vi "20170425-lecture4-1 string.vi"() -> ()   [LabVIEW 2014]
panel:
  out "before substring":string
  out "string 3":string
  out "+/-":string
  out "string 2":string
  out "detected '+' in string":bool
  in  "string":string="Volts DC-1.2312;"
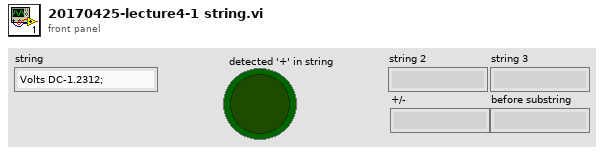
[diagram p1: front panel]
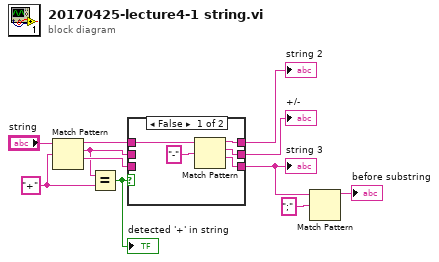
[diagram p0: block diagram]
diagram:
  w11 = "+" ("regular expression")
  n1 = Match Pattern(string="string", regular expression=w11) -> (before substring=w3:string, match substring=w6:string, after substring=w7:string)  [unwired: 1 in, 1 out]
  n2 = Equal?(x=w6, y=w11) -> (x = y?=w10:bool)
  "detected '+' in string" <- w10
  n3 = case shown="False" w10 {
    tunnel: w6 -> [_ w19]
    tunnel: [w15 w17] -> w9
    tunnel: [w14 w19] -> w8
    tunnel: [w13 w18] -> w5
    tunnel: w7 -> [_ w18]
    tunnel: w3 -> [w12 w17]
    frame False {
      n4 = Match Pattern(string=w12, regular expression="-") -> (before substring=w15:string, match substring=w14:string, after substring=w13:string)  [unwired: 1 in, 1 out]
    }
    frame True {
    }
  }
  "string 2" <- w9
  "+/-" <- w8
  "string 3" <- w5
  n5 = Match Pattern(string=w5, regular expression=";") -> (before substring=→"before substring":string)  [unwired: 1 in, 3 out]
